vi "Write Local Port.vi"(8 "error in (no error)":errorcluster, 10 "Local Port":u16, 11 "UDP in":refnum<class "UDP.lvclass">) -> (0 "error out":errorcluster, 3 "UDP out":refnum<class "UDP.lvclass">)   [LabVIEW 2023, in "Protocols.lvlib" / "UDP.lvclass"]
uses:
  UDP.lvclass
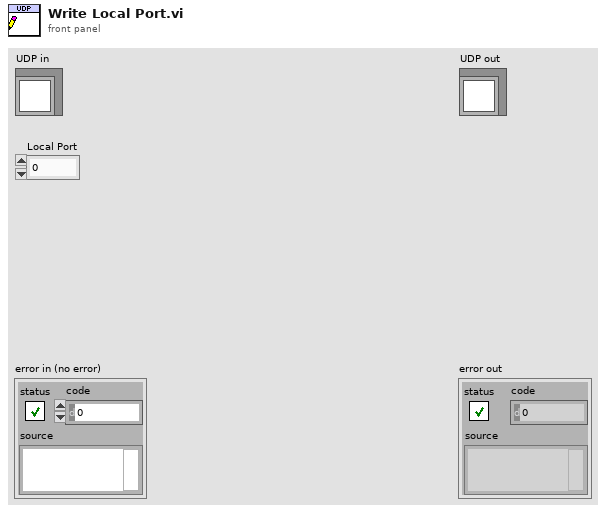
[diagram p1: front panel]
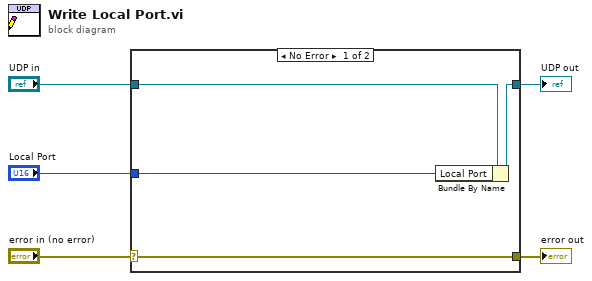
[diagram p0: block diagram]
diagram:
  n1 = case shown="No Error" "error in (no error)" {
    selector: "error in (no error)" -> [w9 w10]
    tunnel: [w9 w10] -> w4
    tunnel: [w7 w11] -> w2
    tunnel: "UDP in" -> [w8 w11]
    tunnel: "Local Port" -> [w6 _]
    frame No Error {
      n2 = Bundle By Name(cluster=w8, "Local Port"=w6) -> (w7:refnum<class "UDP.lvclass">)
    }
    frame Error {
    }
  }
  "error out" <- w4
  "UDP out" <- w2
